vi "Mapping v10.6.3.vi"(5 "Simulate Spectra":bool, 7 "Simulate Drive":bool) -> ()   [LabVIEW 2010]
uses:
  TypeDefs/Mapping Spectra Params.ctl
  TypeDefs/Mapping Drive Params v10.6.0.ctl
  NPC3SG/TypeDefs/NPC3SG Set Positions.ctl
  NPC3SG/TypeDefs/NPC3SG Current Values.ctl
  iHR550/TypeDefs/iHR Current Values.ctl
  ITC503/TypeDefs/ITC503 Current Values.ctl
  TypeDefs/Mapping Input Parameters v10.6.2.ctl
  Symphony/TypeDefs/Symphony Area Format.ctl
  <vilib>/Utility/miscctls.llb/LVPointTypeDef.ctl
  Global Variables.vi
panel:
  in  "Input Parameters":T1={"Drive Connection Port"="", "ITC503 Current Values"={"ITC503 Heater"=0.0, "ITC503 Temperature"=0.0, "ITC503 P"=0.0, "ITC503 I"=0.0, "ITC503 D"=0.0, "ITC503 Setpoint"=0.0, "ITC503 Gradient"=0.0, "ITC503 Heater Auto"=FALSE, "ITC503 PID Auto"=FALSE}, "Wavelengths (nm)"=[], "Drive Current Values"={"Drive X Position"=0.0, "Drive Y Position"=0.0, "Drive Z Position"=0.0}, "iHR Current Values"={"iHR 550 Front Entrance"=0.0, "iHR550 Side Exit"=0.0, "iHR550 Wavelength"=897.9988, "iHR550 Exit Mirror"=2, "iHR550 Grating"="1", "Grating Index"=1}, "Spectra Settings"={"Integration Time"=1.0, "Repetitions"=1, "Mapping Spectra"=TRUE}, "CCD3500 Temperature"=0.0, "Simulate Drive"=FALSE, "Simulate Spectra"=FALSE, "JYCCDLib.IJYCCDReqd"=refnum, "CCD Area"={"XStart"=1, "YStart"=1, "XStop"=2048, "YStop"=512, "XBin"=1, "YBin"=1}, "CCD Gain"=1, "CCD ADC"=0, "Drive Calibration"=path ""} {"CCD ADC" items=["20 kHz       ", " 1 MHz       ", " 1 MHz Ultra ", "500 kHz Wrap"]; "CCD Gain" items=["High Light", "Best Dynamic Range", "High Sensitivity"]; "ITC503 Current Values"."ITC503 Gradient" format="%.2f"; "ITC503 Current Values"."ITC503 Setpoint" min=-273.0 max=300000.0 step=0.0001 format="%.1f"; "ITC503 Current Values"."ITC503 I" format="%_1f"; "ITC503 Current Values"."ITC503 P" format="%_1f"; "ITC503 Current Values"."ITC503 Temperature" min=0.0 max=1645.0 step=1e-05 format="%.2f"; "ITC503 Current Values"."ITC503 Heater" min=0.0 max=100.0 step=0.01 scale=0.0..100.0; "Drive Current Values"."Drive Z Position" min=-273.0 max=300000.0 step=0.0001 format="%.3f"; "Drive Current Values"."Drive Y Position" min=-273.0 max=300000.0 step=0.0001 format="%.3f"; "Drive Current Values"."Drive X Position" min=-273.0 max=300000.0 step=0.0001 format="%.3f"; "iHR Current Values"."iHR550 Exit Mirror" items=["EntranceMirror", "ExitMirror", "Front", "Side"]; "Spectra Settings"."Repetitions" min=1 max=100 step=1; "Spectra Settings"."Integration Time" min=0.5 max=6000.0 step=1.0 format="%.1f"}
  out "JYCCDLib.IJYCCDReqd":refnum<k7>
  out "AutoClose":bool
  out "ITC503 Temperature":dbl caption="Sample (K)" min=10.0 max=160.0 step=0.1 format="%.3f"
  out "CCD3500 Temperature":dbl caption="CCD (°C)" min=10.0 max=160.0 step=0.1 format="%.1f"
  in  "CCD Current Rep.":string="0/0"
  in  "Pause":bool
  out "Current Position":T3 {"Drive Z Position" min=-273.0 max=300000.0 step=0.0001 format="%.3f"; "Drive Y Position" min=-273.0 max=300000.0 step=0.0001 format="%.3f"; "Drive X Position" min=-273.0 max=300000.0 step=0.0001 format="%.3f"}
  out "Target Position":T7={"Drive X Set"=10.0, "Drive Y Set"=10.0, "Drive Z Set"=10.0} {"Drive X Set" min=10.0 max=160.0 step=0.1 format="%.3f"; "Drive Z Set" min=10.0 max=160.0 step=0.1 format="%.3f"; "Drive Y Set" min=10.0 max=160.0 step=0.1 format="%.3f"}
  out "Progress":u8(slide) max=10 scale=0.0..100.0
  out "Objective Running":bool caption="Obj."
  out "CCD Running":bool caption="CCD"
  in  "Save Map":bool
  in  "Spectra Params":T5={"Integration Time"=10.0, "Repetitions"=10, "Mapping Spectra"=TRUE} {"Repetitions" min=1 max=100 step=1; "Integration Time" min=0.5 max=6000.0 step=1.0 format="%.1f"}
  in  "Drive Settings":refnum<visa-resource-name>
  in  "Z Position":dbl caption="Z (µm)" min=0.0 max=100.0 step=0.1 format="%.1f"
  in  "Mapping Params":T8={"X Start Position"=0.0, "X Stop Position"=10.0, "Y Start Position"=0.0, "Y Stop Position"=10.0, "Step Size"=1.0} {"Step Size" min=0.005 max=20.0 step=0.005 format="%.3f"; "Y Stop Position" min=0.0 max=140.0 step=0.005 format="%.3f"; "Y Start Position" min=0.0 max=140.0 step=0.005 format="%.3f"; "X Stop Position" min=0.0 max=140.0 step=0.005 format="%.3f"; "X Start Position" min=0.0 max=140.0 step=0.005 format="%.3f"}
  in  "Exit":bool
  out "Measuring":bool
  in  "Start":bool
  out "Filename":string
  out "Full Data":dbl[][](array[numeric])
  out "Live Data":dbl[][](array[numeric])
  in  "ITC503 Current Values":T2 {"ITC503 Gradient" format="%.2f"; "ITC503 Setpoint" min=-273.0 max=300000.0 step=0.0001 format="%.1f"; "ITC503 I" format="%_1f"; "ITC503 P" format="%_1f"; "ITC503 Temperature" min=0.0 max=1645.0 step=1e-05 format="%.2f"; "ITC503 Heater" min=0.0 max=100.0 step=0.01 scale=0.0..100.0}
  in  "iHR Current Values":T4={"iHR 550 Front Entrance"=0.0, "iHR550 Side Exit"=0.0, "iHR550 Wavelength"=897.9988, "iHR550 Exit Mirror"=2, "iHR550 Grating"="1", "Grating Index"=1} {"iHR550 Exit Mirror" items=["EntranceMirror", "ExitMirror", "Front", "Side"]}
  in  "Wavelengths (nm)":dbl[](array[numeric])
  # "Status"
  # "Active"
  # "Target"
  # "Current"
  # "Parameters"
  # "Spectral"
  # "Spectral / Video Mapping"
  # "Mapping"
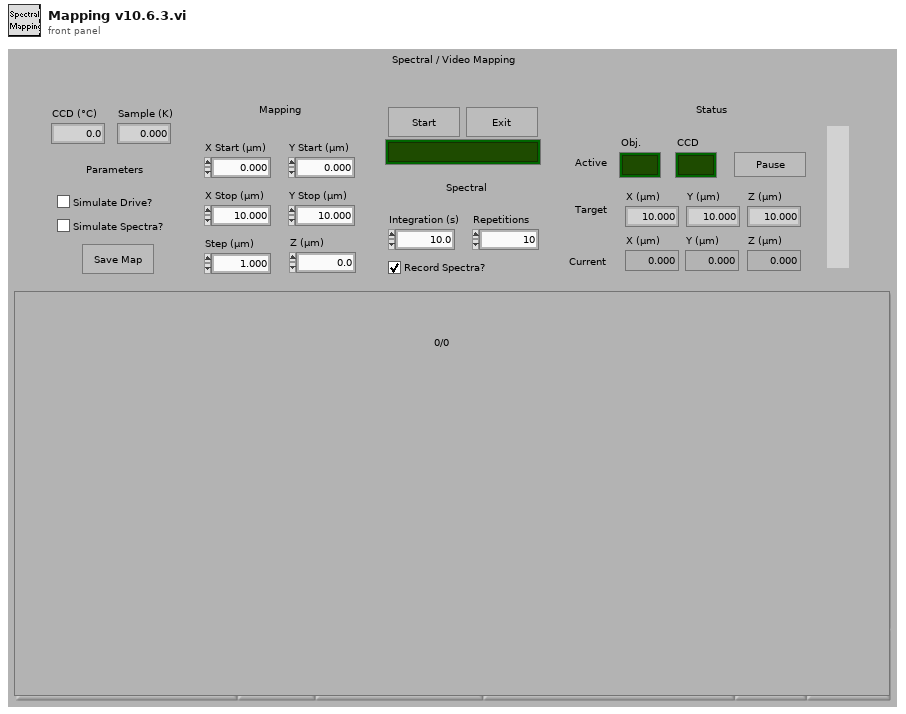
[diagram p1: front panel]
types:
  T1 = typedef "Mapping Input Parameters v10.6.2.ctl" = cluster{"Drive Connection Port":refnum<visa-resource-name>, "ITC503 Current Values":T2, "Wavelengths (nm)":dbl[], "Drive Current Values":T3, "iHR Current Values":T4, "Spectra Settings":T5, "CCD3500 Temperature":dbl, "Simulate Drive":bool, "Simulate Spectra":bool, "JYCCDLib.IJYCCDReqd":refnum<k7>, "CCD Area":T6, "CCD Gain":u16, "CCD ADC":u16, "Drive Calibration":path}
  T2 = typedef "ITC503 Current Values.ctl" = cluster{"ITC503 Heater":dbl, "ITC503 Temperature":dbl, "ITC503 P":dbl, "ITC503 I":dbl, "ITC503 D":dbl, "ITC503 Setpoint":dbl, "ITC503 Gradient":dbl, "ITC503 Heater Auto":bool, "ITC503 PID Auto":bool}
  T3 = typedef "NPC3SG Current Values.ctl" = cluster{"Drive X Position":dbl, "Drive Y Position":dbl, "Drive Z Position":dbl}
  T4 = typedef "iHR Current Values.ctl" = cluster{"iHR 550 Front Entrance":dbl, "iHR550 Side Exit":dbl, "iHR550 Wavelength":dbl, "iHR550 Exit Mirror":i32, "iHR550 Grating":string, "Grating Index":i32}
  T5 = typedef "Mapping Spectra Params.ctl" = cluster{"Integration Time":dbl, "Repetitions":u16, "Mapping Spectra":bool}
  T6 = typedef "Symphony Area Format.ctl" = cluster{"XStart":i32, "YStart":i32, "XStop":i32, "YStop":i32, "XBin":i32, "YBin":i32}
  T7 = typedef "NPC3SG Set Positions.ctl" = cluster{"Drive X Set":dbl, "Drive Y Set":dbl, "Drive Z Set":dbl}
  T8 = typedef "Mapping Drive Params v10.6.0.ctl" = cluster{"X Start Position":dbl, "X Stop Position":dbl, "Y Start Position":dbl, "Y Stop Position":dbl, "Step Size":dbl}
  T9 = typedef "LVPointTypeDef.ctl" = cluster{"Horizontal":i16, "Vertical":i16}
  T10 = cluster{"Intensities":dbl[], "Wavelengths":dbl[]}[]
  T11 = cluster{"Intensities":dbl[], "Wavelengths":dbl[]}
  T12 = enum32{"invalid app kind", "Development System", "Run Time System", "Student Edition", "Embedded LabVIEW", "Evaluation", "Custom"}
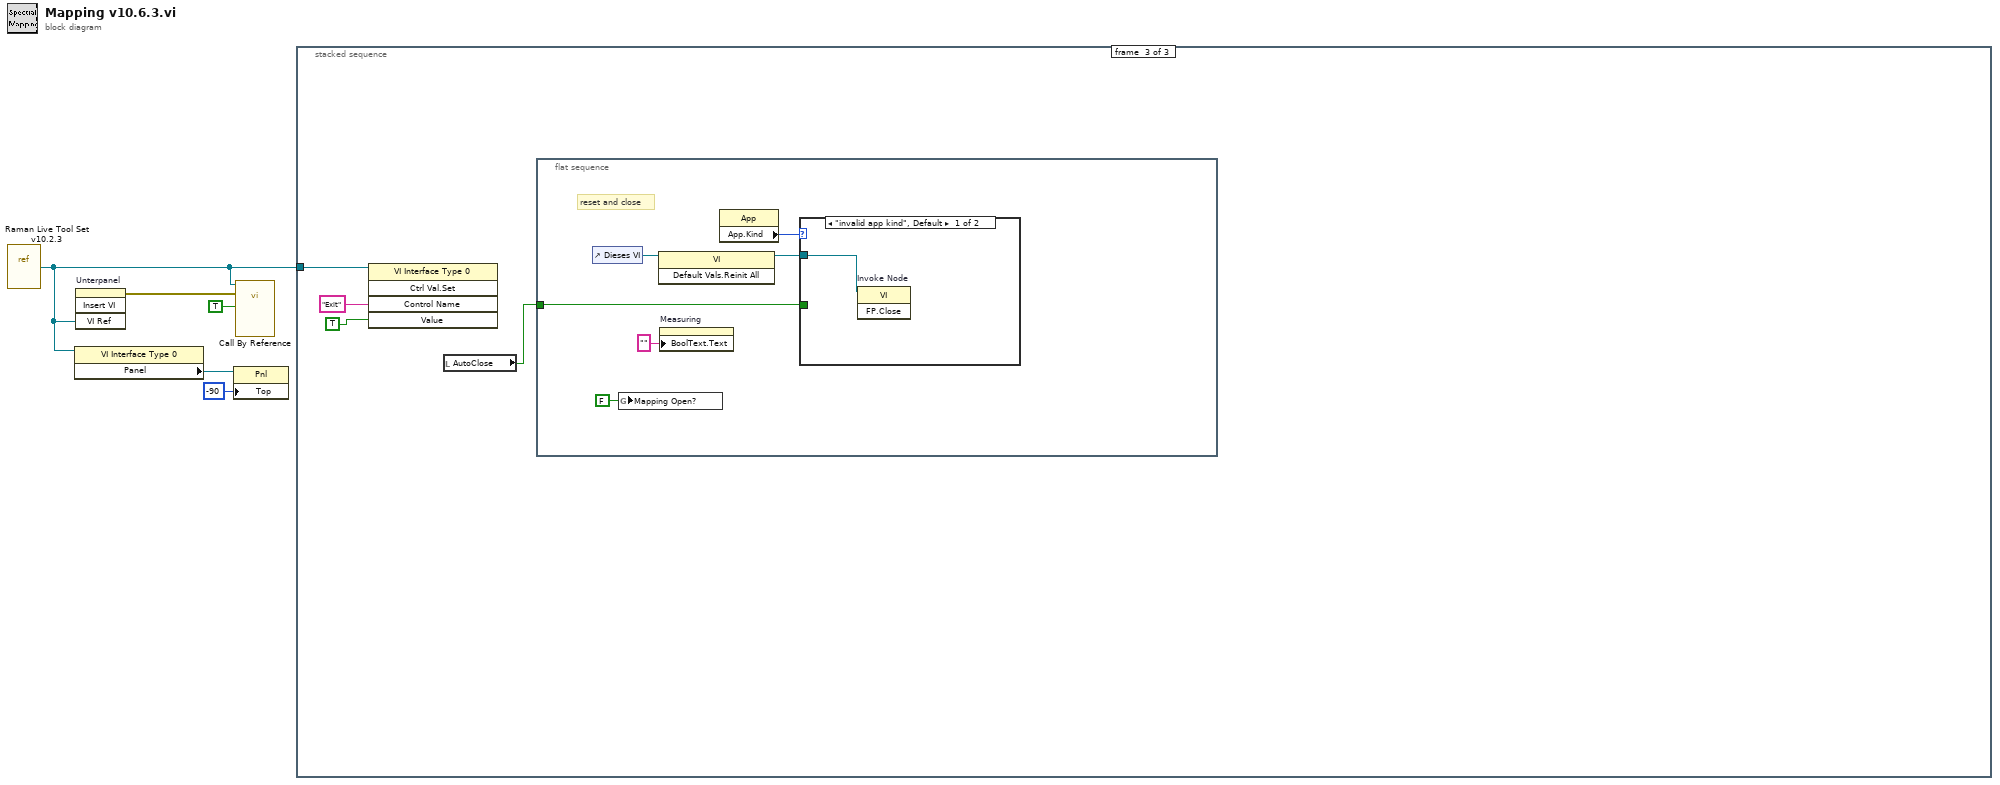
[diagram p0: block diagram]
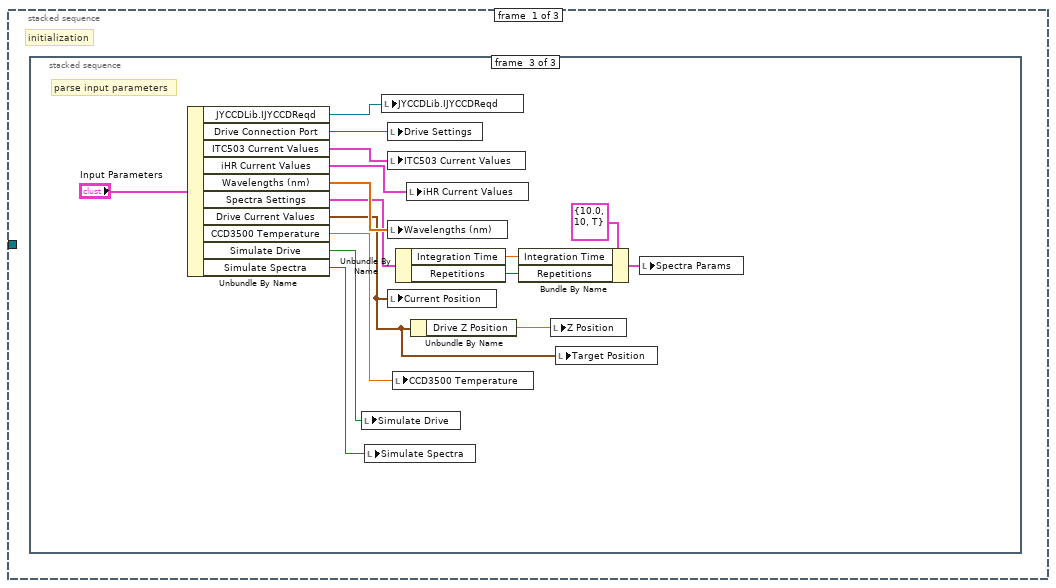
[diagram p2: hidden frame]
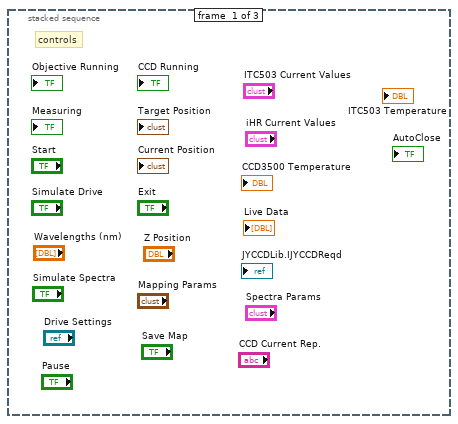
[diagram p3: hidden frame]
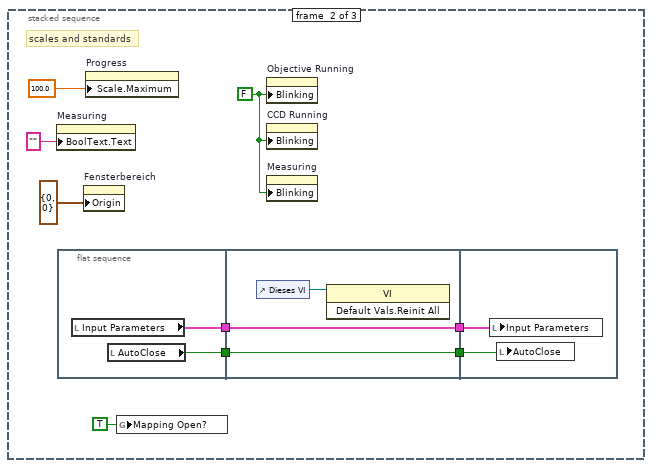
[diagram p4: hidden frame]
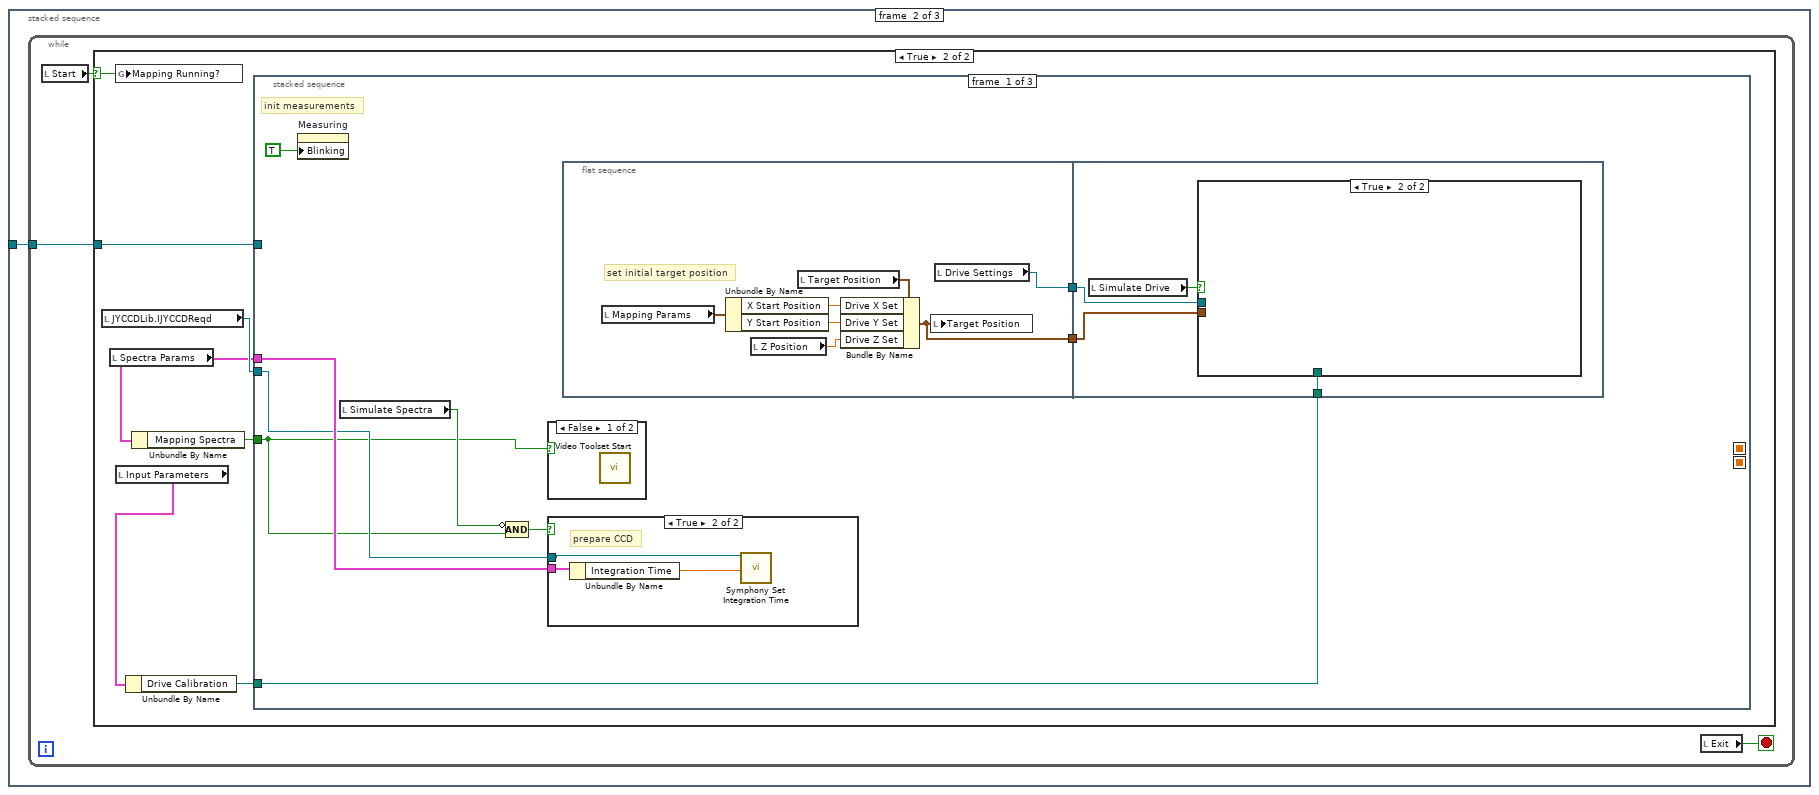
[diagram p5: hidden frame]
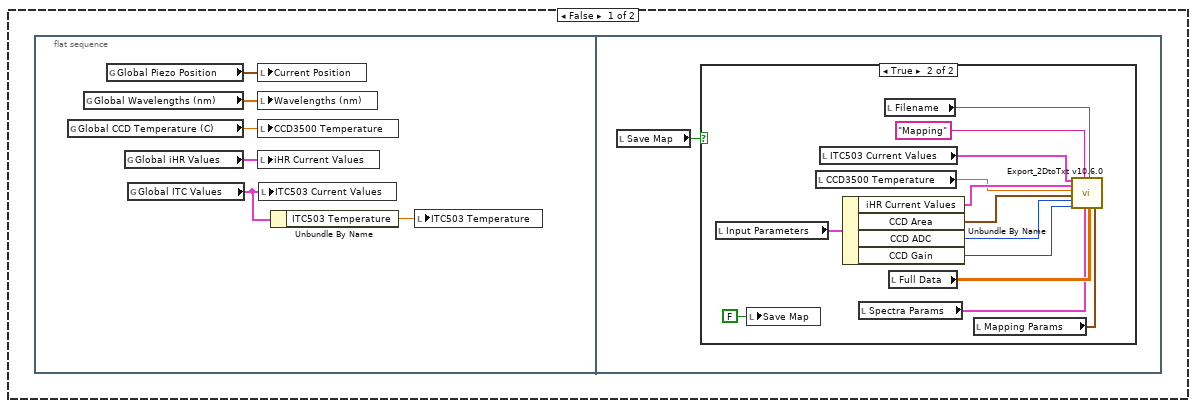
[diagram p6: hidden frame]
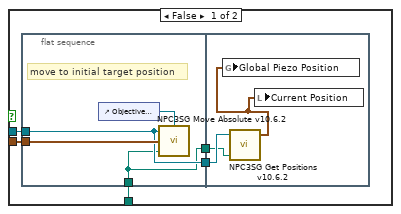
[diagram p10: hidden frame]
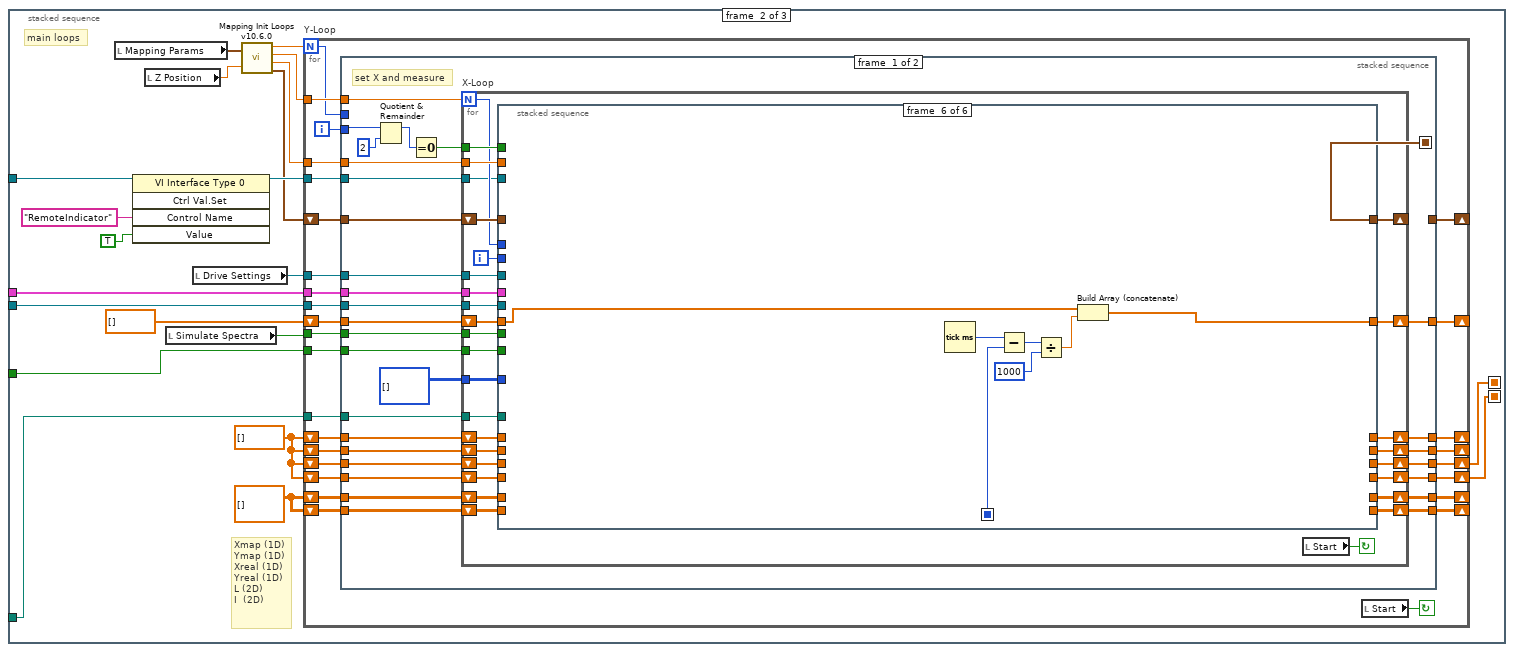
[diagram p11: hidden frame]
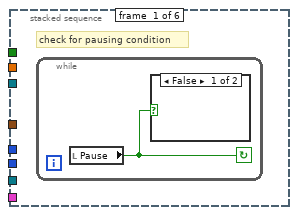
[diagram p12: hidden frame]
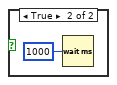
[diagram p13: hidden frame]
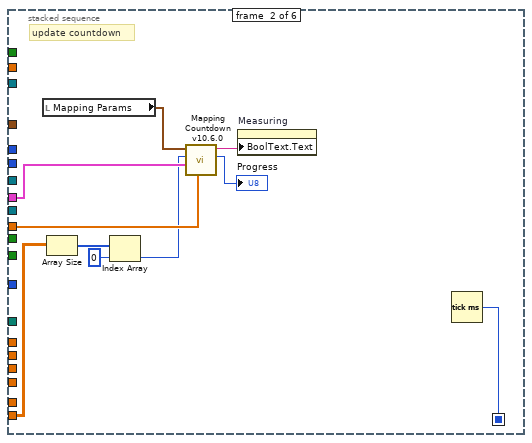
[diagram p14: hidden frame]
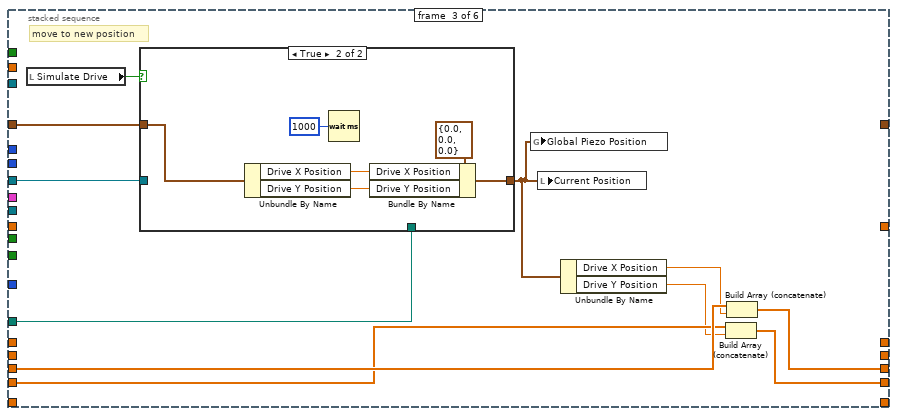
[diagram p15: hidden frame]
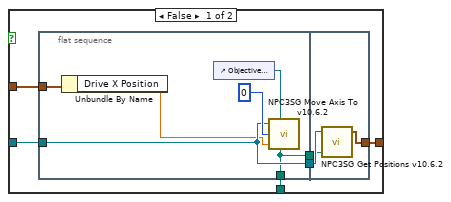
[diagram p16: hidden frame]
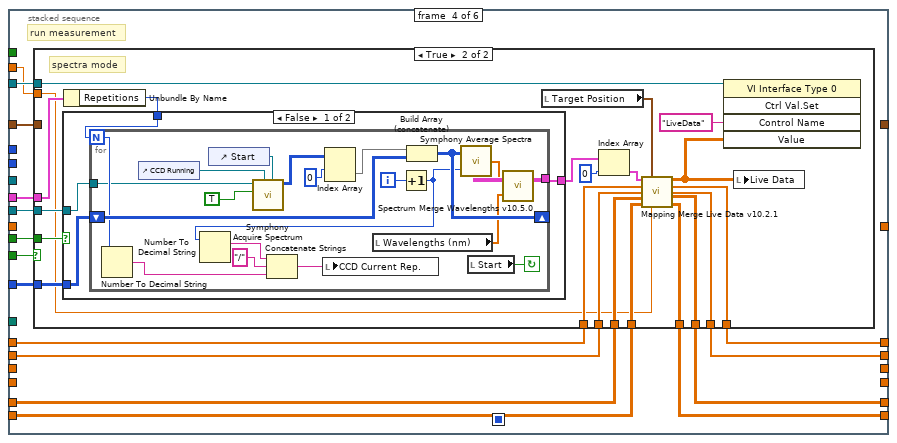
[diagram p17: hidden frame]
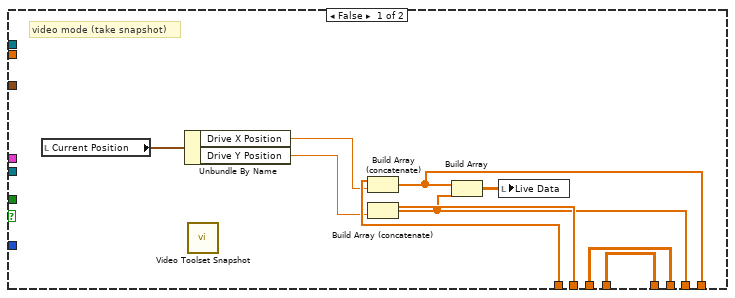
[diagram p18: hidden frame]
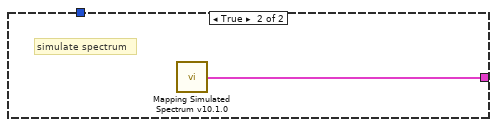
[diagram p19: hidden frame]
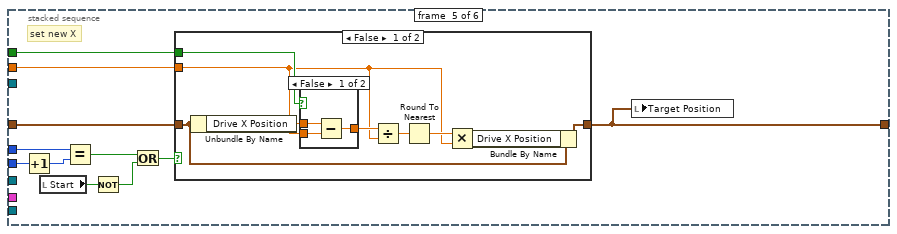
[diagram p20: hidden frame]
diagram:
  n1 = vi-ref "Raman Live Tool Set v10.2.3.vi"() -> (w3:refnum<vi>)
  n2 = property class="VI Interface Type 0"(reference=w3) -> ("Panel"=w2:refnum<vi>)  [unwired: 1 in, 2 out]
  n3 = invoke on="Unterpanel" class="Unterpanel" method="Insert VI"("VI Ref"=w3) -> (error out=w5:errorcluster)  [unwired: 3 in, 3 out]
  n4 = property class="Pnl"(reference=w2, "Top"=-90 ("Position:Oben")) -> ()  [unwired: 1 in, 2 out]
  n5 = call-by-ref "?"(reference=w3, error in=w5, "RemoteIndicator"=TRUE) -> ()  [unwired: 3 in, 2 out]
  n6 = stacked-sequence {
    tunnel: w3 -> [_ w38 w425]
    frame #0 {
      # "initialization"
      n7 = stacked-sequence {
        frame #0 {
          # "controls"
        }
        frame #1 {
          w12 = FALSE ("Blinkend")
          # "scales and standards"
          n8 = property on="Measuring" class="Bool (strict)"("BoolText.Text"="" ("Boolescher Text.Text")) -> ()  [unwired: 2 in, 2 out]
          n9 = flat-sequence {
            tunnel: [w16] -> w9
            tunnel: [w15] -> w6
            tunnel: [w18] -> w10
            tunnel: w9 -> [w18]
            tunnel: [w17] -> w7
            tunnel: w6 -> [w17]
            tunnel: w10 -> [w21]
            tunnel: w7 -> [w20]
            frame #0 {
              n10 = local read "Input Parameters"() -> (w16:T1)
              n11 = local read "AutoClose"() -> (w15:bool)
            }
            frame #1 {
              n12 = control-ref of="Dieses VI"() -> (w19:refnum<vi>)
              n13 = invoke class="VI" method="Default Vals.Reinit All"(reference=w19) -> ()  [unwired: 2 in, 3 out]
            }
            frame #2 {
              n14 = local write "Input Parameters"(w21) -> ()
              n15 = local write "AutoClose"(w20) -> ()
            }
          }
          n16 = property on="Fensterbereich" class="Pane"("Origin"=T9 {"Horizontal"=0, "Vertical"=0}) -> ()  [unwired: 2 in, 2 out]
          n17 = property on="Progress" class="Slide (strict)"("Scale.Maximum"=100.0 ("Skalierung.Bereich:Maximum")) -> ()  [unwired: 2 in, 2 out]
          n18 = global write "Global Variables.vi" "Mapping Open?"(TRUE ("Mapping Open?")) -> ()
          n19 = property on="Objective Running" class="Bool (strict)"("Blinking"=w12) -> ()  [unwired: 2 in, 2 out]
          n20 = property on="CCD Running" class="Bool (strict)"("Blinking"=w12) -> ()  [unwired: 2 in, 2 out]
          n21 = property on="Measuring" class="Bool (strict)"("Blinking"=w12) -> ()  [unwired: 2 in, 2 out]
        }
        frame #2 {
          # "parse input parameters"
          n22 = Unbundle By Name("Input Parameters") -> ("JYCCDLib.IJYCCDReqd"=w24:refnum<k7>, "Drive Connection Port"=w36:refnum<visa-resource-name>, "ITC503 Current Values"=w37:T2, "iHR Current Values"=w27:T4, "Wavelengths (nm)"=w35:dbl[], "Spectra Settings"=w33:T5, "Drive Current Values"=w22:T3, "CCD3500 Temperature"=w28:dbl, "Simulate Drive"=w26:bool, "Simulate Spectra"=w25:bool)
          n23 = local write "Simulate Drive"(w26) -> ()
          n24 = local write "Simulate Spectra"(w25) -> ()
          n25 = local write "JYCCDLib.IJYCCDReqd"(w24) -> ()
          n26 = local write "Drive Settings"(w36) -> ()
          n27 = local write "ITC503 Current Values"(w37) -> ()
          n28 = local write "Wavelengths (nm)"(w35) -> ()
          n29 = local write "Current Position"(w22) -> ()
          n30 = local write "CCD3500 Temperature"(w28) -> ()
          n31 = Unbundle By Name(w33) -> ("Integration Time"=w31:dbl, "Repetitions"=w30:u16)
          n32 = local write "iHR Current Values"(w27) -> ()
          n33 = Unbundle By Name(w22) -> ("Drive Z Position"=w34:dbl)
          n34 = Bundle By Name(cluster=T5 {"Integration Time"=10.0, "Repetitions"=10, "Mapping Spectra"=TRUE} ("Mapping Spectra Settings"), "Integration Time"=w31, "Repetitions"=w30) -> (w29:T5)
          n35 = local write "Z Position"(w34) -> ()
          n36 = local write "Target Position"(w22) -> ()
          n37 = local write "Spectra Params"(w29) -> ()
        }
      }
    }
    frame #1 {
      n38 = while {
        tunnel: w38 -> [w41]
        stop <- w40 stop-if-true
        n39 = local read "Start"() -> (w39:bool)
        n40 = case shown="True" w39 {
          selector: w39 -> [_ w65]
          tunnel: w41 -> [_ w68]
          frame False {
            n41 = flat-sequence {
              frame #0 {
                n42 = global read "Global Variables.vi" "Global CCD Temperature (C)"() -> (w47:dbl)
                n43 = global read "Global Variables.vi" "Global Wavelengths (nm)"() -> (w45:dbl[])
                n44 = global read "Global Variables.vi" "Global Piezo Position"() -> (w46:T3)
                n45 = global read "Global Variables.vi" "Global iHR Values"() -> (w44:T4)
                n46 = global read "Global Variables.vi" "Global ITC Values"() -> (w43:T2)
                n47 = local write "Current Position"(w46) -> ()
                n48 = local write "Wavelengths (nm)"(w45) -> ()
                n49 = local write "CCD3500 Temperature"(w47) -> ()
                n50 = local write "iHR Current Values"(w44) -> ()
                n51 = local write "ITC503 Current Values"(w43) -> ()
                n52 = Unbundle By Name(w43) -> ("ITC503 Temperature"=w42:dbl)
                n53 = local write "ITC503 Temperature"(w42) -> ()
              }
              frame #1 {
                n54 = local read "Save Map"() -> (w48:bool)
                n55 = case shown="True" w48 {
                  frame False {
                  }
                  frame True {
                    n56 = local read "Input Parameters"() -> (w57:T1)
                    n57 = local write "Save Map"(FALSE ("Save Map")) -> ()
                    n58 = local read "CCD3500 Temperature"() -> (w51:dbl)
                    n59 = local read "ITC503 Current Values"() -> (w54:T2)
                    n60 = Unbundle By Name(w57) -> ("iHR Current Values"=w52:T4, "CCD Area"=w53:T6, "CCD ADC"=w56:u16, "CCD Gain"=w55:u16)
                    n61 = local read "Spectra Params"() -> (w50:T5)
                    n62 = local read "Filename"() -> (w60:string)
                    n63 = local read "Full Data"() -> (w58:dbl[][])
                    n64 = local read "Mapping Params"() -> (w49:T8)
                    n65 = call "Export_2DtoTxt v10.6.0.vi"("ITC503 Current Values"=w54, "iHR Current Values"=w52, "CCD Temperature"=w51, "CCD Area"=w53, "CCD ADC"=w56, "CCD Gain"=w55, "Export Type"="Mapping", "Spectra Settings"=w50, "Filename"=w60, "Data (2D)"=w58, "Mapping Parameters"=w49) -> ()  [unwired: 8 in, 1 out]
                  }
                }
              }
            }
          }
          frame True {
            n66 = local read "JYCCDLib.IJYCCDReqd"() -> (w67:refnum<k7>)
            n67 = local read "Spectra Params"() -> (w66:T5)
            n68 = global write "Global Variables.vi" "Mapping Running?"(w65) -> ()
            n69 = local read "Input Parameters"() -> (w63:T1)
            n70 = Unbundle By Name(w63) -> ("Drive Calibration"=w62:path)
            n71 = Unbundle By Name(w66) -> ("Mapping Spectra"=w64:bool)
            n72 = stacked-sequence {
              seq-local: [_ w105 _] -> [_ _ w400]
              seq-local: [_ w106 _] -> [_ _ w399]
              tunnel: w68 -> [_ w116 _]
              tunnel: w64 -> [w70 w115 w401]
              tunnel: w66 -> [w72 w113 _]
              tunnel: w67 -> [w71 w112 _]
              tunnel: w62 -> [w69 w104 _]
              frame #0 {
                # "init measurements"
                n73 = property on="Measuring" class="Bool (strict)"("Blinking"=TRUE ("Blinkend")) -> ()  [unwired: 2 in, 2 out]
                n74 = local read "Simulate Spectra"() -> (w74:bool)
                n75 = Compound Arithmetic op=AND(invert w74, w70) -> (w73:bool)
                n76 = case shown="False" w70 {
                  frame False {
                    n77 = call "Video Toolset Start.vi"() -> ()  [unwired: 3 in]
                  }
                  frame True {
                  }
                }
                n78 = case shown="True" w73 {
                  tunnel: w71 -> [_ w80]
                  tunnel: w72 -> [_ w79]
                  frame False {
                  }
                  frame True {
                    # "prepare CCD"
                    n79 = Unbundle By Name(w79) -> ("Integration Time"=w78:dbl)
                    n80 = call "Symphony Set Integration Time.vi"("JYCCDLib.IJYCCDReqd"=w80, "Integration (s)"=w78) -> ()  [unwired: 13 in, 1 out]
                  }
                }
                n81 = flat-sequence {
                  tunnel: [w82] -> w76
                  tunnel: [w81] -> w75
                  tunnel: w76 -> [w89]
                  tunnel: w75 -> [w90]
                  tunnel: w69 -> [w88]
                  frame #0 {
                    # "set initial target position"
                    n82 = local read "Mapping Params"() -> (w87:T8)
                    n83 = Unbundle By Name(w87) -> ("X Start Position"=w85:dbl, "Y Start Position"=w84:dbl)
                    n84 = local read "Z Position"() -> (w83:dbl)
                    n85 = local read "Target Position"() -> (w86:T7)
                    n86 = Bundle By Name(cluster=w86, "Drive X Set"=w85, "Drive Y Set"=w84, "Drive Z Set"=w83) -> (w82:T7)
                    n87 = local write "Target Position"(w82) -> ()
                    n88 = local read "Drive Settings"() -> (w81:refnum<visa-resource-name>)
                  }
                  frame #1 {
                    n89 = local read "Simulate Drive"() -> (w91:bool)
                    n90 = case shown="True" w91 {
                      tunnel: w90 -> [w96 _]
                      tunnel: w89 -> [w94 _]
                      tunnel: w88 -> [w93 _]
                      frame False {
                        n91 = flat-sequence {
                          tunnel: w96 -> [w98]
                          tunnel: [w98] -> w95
                          tunnel: w94 -> [w99]
                          tunnel: w93 -> [w97]
                          tunnel: [w97] -> w92
                          tunnel: w95 -> [w102]
                          tunnel: w92 -> [w101]
                          frame #0 {
                            # "move to initial target position"
                            n92 = control-ref of="Objective Running"() -> (w100:refnum<vi>)
                            n93 = call "NPC3SG Move Absolute v10.6.2.vi"("Running"=w100, "Calibration File"=w97, "Drive New Abs. Positions"=w99, "Drive Visa Name"=w98) -> ()  [unwired: 1 in]
                          }
                          frame #1 {
                            n94 = call "NPC3SG Get Positions v10.6.2.vi"("Drive Visa Name"=w102, "Calibration File"=w101) -> ("Drive Current Values"=w103:T3)  [unwired: 5 in]
                            n95 = global write "Global Variables.vi" "Global Piezo Position"(w103) -> ()
                            n96 = local write "Current Position"(w103) -> ()
                          }
                        }
                      }
                      frame True {
                      }
                    }
                  }
                }
              }
              frame #1 {
                w124 = dbl[][] []
                w107 = dbl[] []
                # "main loops"
                # "Xmap (1D)\nYmap (1D)\nXreal (1D)\nYreal (1D)\nL (2D)\nI  (2D)"
                n97 = local read "Mapping Params"() -> (w110:T8)
                n98 = invoke class="VI Interface Type 0" method="Ctrl Val.Set"(reference=w116, "Control Name"="RemoteIndicator" ("Elementname"), "Value"=TRUE) -> (reference out=w118:refnum<vi>)  [unwired: 2 in, 4 out]
                n99 = local read "Z Position"() -> (w109:dbl)
                n100 = local read "Simulate Spectra"() -> (w108:bool)
                n101 = local read "Drive Settings"() -> (w111:refnum<visa-resource-name>)
                n102 = call "Mapping Init Loops v10.6.0.vi"("Z Position"=w109, "Mapping Params"=w110) -> ("Start Positions"=w117:T3, "Step Size"=w119:dbl, "X Steps"=w120:dbl, "Y Steps"=w121:dbl)
                n103 = for "Y-Loop" {
                  N: w121 -> [w138]
                  tunnel: w120 -> [w151]
                  tunnel: w119 -> [w150]
                  shift-right: [w136] -> _
                  shift-left: w117 -> [w137]
                  shift-right: [w142] -> _
                  shift-left: w124 -> [w146]
                  shift-right: [w143] -> _
                  shift-left: w124 -> [w147]
                  shift-right: [w145] -> _
                  shift-left: w107 -> [w149]
                  shift-right: [w144] -> _
                  shift-left: w107 -> [w148]
                  tunnel: w118 -> [w140]
                  tunnel: w108 -> [w139]
                  tunnel: w111 -> [w135]
                  tunnel: w115 -> [w134]
                  tunnel: w113 -> [w133]
                  shift-right: [w131] -> _
                  shift-left: dbl[] [] -> [w132]
                  tunnel: w112 -> [w130]
                  shift-right: [w127] -> w106
                  shift-left: w107 -> [w128]
                  shift-right: [w126] -> w105
                  shift-left: w107 -> [w129]
                  tunnel: w104 -> [w125]
                  i -> [w141]
                  stop <- w152 continue-if-true
                  n104 = stacked-sequence {
                    seq-local: [w167 _] -> [_ w370]
                    tunnel: w151 -> [w182 _]
                    tunnel: w150 -> [w181 w371]
                    tunnel: w149 -> [w180 _]
                    tunnel: w148 -> [w179 _]
                    tunnel: w147 -> [w178 _]
                    tunnel: w146 -> [w154 _]
                    tunnel: [w177 _] -> w145
                    tunnel: [w176 _] -> w144
                    tunnel: [w175 _] -> w143
                    tunnel: [w174 _] -> w142
                    tunnel: w141 -> [w171 w374]
                    tunnel: w140 -> [w169 _]
                    tunnel: w139 -> [w168 _]
                    tunnel: w138 -> [_ w372]
                    tunnel: w137 -> [w166 _]
                    tunnel: [_ w368] -> w136
                    tunnel: w135 -> [w165 w369]
                    tunnel: w134 -> [w164 _]
                    tunnel: w133 -> [w163 _]
                    tunnel: w132 -> [w162 _]
                    tunnel: [w161 _] -> w131
                    tunnel: w130 -> [w160 _]
                    tunnel: w129 -> [w158 _]
                    tunnel: w128 -> [w157 _]
                    tunnel: [w156 _] -> w127
                    tunnel: [w155 _] -> w126
                    tunnel: w125 -> [w153 w362]
                    frame #0 {
                      # "set X and measure"
                      n105 = Quotient & Remainder(x=w171, y=2) -> (x-y*floor(x/y)=w172:i32)  [unwired: 1 out]
                      n106 = Equal To 0?(x=w172) -> (x = 0?=w170:bool)
                      n107 = for "X-Loop" {
                        N: w182 -> [w197]
                        tunnel: w181 -> [w209]
                        shift-right: [w208] -> w167
                        shift-left: w166 -> [w210]
                        shift-right: [w203] -> w177
                        shift-left: w180 -> [w207]
                        shift-right: [w202] -> w176
                        shift-left: w179 -> [w206]
                        shift-right: [w200] -> w175
                        shift-left: w178 -> [w205]
                        shift-right: [w201] -> w174
                        shift-left: w154 -> [w204]
                        tunnel: w170 -> [w199]
                        tunnel: w169 -> [w196]
                        tunnel: w168 -> [w195]
                        tunnel: w165 -> [w194]
                        tunnel: w164 -> [w193]
                        tunnel: w163 -> [w192]
                        shift-right: [w191] -> w161
                        shift-left: w162 -> [w190]
                        tunnel: w160 -> [w189]
                        tunnel: u16[][] [] -> [w188]
                        shift-right: [w184] -> w155
                        shift-left: w158 -> [w187]
                        shift-right: [w185] -> w156
                        shift-left: w157 -> [w186]
                        tunnel: w153 -> [w183]
                        i -> [w198]
                        stop <- w211 continue-if-true
                        n108 = stacked-sequence {
                          seq-local: [_ w218 _ _ _ _] -> [_ _ _ _ _ w358]
                          tunnel: w210 -> [_ _ w234 w271 w335 _]
                          tunnel: w209 -> [_ _ _ w256 w333 _]
                          tunnel: [_ _ _ _ w332 _] -> w208
                          tunnel: w207 -> [_ _ _ w270 _ _]
                          tunnel: w206 -> [_ _ _ w269 _ _]
                          tunnel: w205 -> [_ _ _ w267 _ _]
                          tunnel: w204 -> [_ w217 _ w268 _ _]
                          tunnel: [_ _ _ w266 _ _] -> w203
                          tunnel: [_ _ _ w265 _ _] -> w202
                          tunnel: [_ _ _ w264 _ _] -> w201
                          tunnel: [_ _ _ w263 _ _] -> w200
                          tunnel: w199 -> [_ _ _ _ w334 _]
                          tunnel: w198 -> [_ _ _ _ w338 _]
                          tunnel: w197 -> [_ _ _ _ w336 _]
                          tunnel: w196 -> [_ _ _ w262 _ _]
                          tunnel: w195 -> [_ _ _ w261 _ _]
                          tunnel: w194 -> [_ _ w232 _ _ _]
                          tunnel: w193 -> [_ _ _ w260 _ _]
                          tunnel: w192 -> [_ w220 _ w258 _ _]
                          tunnel: [_ _ _ _ _ w355] -> w191
                          tunnel: w190 -> [_ w219 _ _ _ w357]
                          tunnel: w189 -> [_ _ _ w259 _ _]
                          tunnel: w188 -> [_ _ _ w257 _ _]
                          tunnel: w187 -> [_ _ w231 _ _ _]
                          tunnel: w186 -> [_ _ w230 _ _ _]
                          tunnel: [_ _ w227 _ _ _] -> w185
                          tunnel: [_ _ w226 _ _ _] -> w184
                          tunnel: w183 -> [_ _ w224 _ _ _]
                          frame #0 {
                            # "check for pausing condition"
                            n109 = while {
                              stop <- w212 continue-if-true
                              n110 = local read "Pause"() -> (w212:bool)
                              n111 = case shown="False" w212 {
                                frame False {
                                }
                                frame True {
                                n112 = Wait (ms)(milliseconds to wait=u32 1000) -> ()  [unwired: 1 out]
                                }
                              }
                            }
                          }
                          frame #1 {
                            # "update countdown"
                            n113 = local read "Mapping Params"() -> (w223:T8)
                            n114 = Array Size(array=w217) -> (size(s)=w216:i32[])
                            n115 = Index Array(array=w216, index=0) -> (element=w214:i32)
                            n116 = call "Mapping Countdown v10.6.0.vi"("Execution Times (s)"=w219, "Mapping Spectra Settings"=w220, "Ready Steps"=w214, "Mapping Drive Parameters"=w223) -> ("Progress"=→"Progress":i16, "Time String"=w221:string)  [unwired: 6 in]
                            n117 = property on="Measuring" class="Bool (strict)"("BoolText.Text"=w221) -> ()  [unwired: 2 in, 2 out]
                            n118 = Tick Count (ms)() -> (millisecond timer value=w218:u32)
                          }
                          frame #2 {
                            # "move to new position"
                            n119 = local read "Simulate Drive"() -> (w233:bool)
                            n120 = case shown="True" w233 {
                              tunnel: w234 -> [w240 w254]
                              tunnel: w232 -> [w239 _]
                              tunnel: [w237 w250] -> w225
                              tunnel: w224 -> [w236 _]
                              frame False {
                                n121 = flat-sequence {
                                tunnel: w240 -> [w243]
                                tunnel: w239 -> [w244]
                                tunnel: [w244] -> w238
                                tunnel: w236 -> [w241]
                                tunnel: [w241] -> w235
                                tunnel: w238 -> [w249]
                                tunnel: [w248] -> w237
                                tunnel: w235 -> [w247]
                                frame #0 {
                                n122 = Unbundle By Name(w243) -> ("Drive X Position"=w242:dbl)
                                n123 = control-ref of="Objective Running"() -> (w245:refnum<vi>)
                                n124 = call "NPC3SG Move Axis To v10.6.2.vi"("Drive Visa Name"=w244, "Running"=w245, "Axis"=0, "Drive Set"=w242, "Calibration File"=w241) -> ()  [unwired: 2 in, 1 out]
                                }
                                frame #1 {
                                n125 = call "NPC3SG Get Positions v10.6.2.vi"("Drive Visa Name"=w249, "Calibration File"=w247) -> ("Drive Current Values"=w248:T3)  [unwired: 5 in]
                                }
                                }
                              }
                              frame True {
                                n126 = Unbundle By Name(w254) -> ("Drive X Position"=w255:dbl, "Drive Y Position"=w252:dbl)
                                n127 = Wait (ms)(milliseconds to wait=u32 1000 ("Zu wartende ms")) -> ()  [unwired: 1 out]
                                n128 = Bundle By Name(cluster=T3 {"Drive X Position"=0.0, "Drive Y Position"=0.0, "Drive Z Position"=0.0} ("Drive Current Values"), "Drive X Position"=w255, "Drive Y Position"=w252) -> (w250:T3)
                              }
                            }
                            n129 = global write "Global Variables.vi" "Global Piezo Position"(w225) -> ()
                            n130 = local write "Current Position"(w225) -> ()
                            n131 = Unbundle By Name(w225) -> ("Drive X Position"=w229:dbl, "Drive Y Position"=w228:dbl)
                            n132 = Build Array (concatenate)(w230, w228) -> (w227:dbl[])
                            n133 = Build Array (concatenate)(w231, w229) -> (w226:dbl[])
                          }
                          frame #3 {
                            # "run measurement"
                            n134 = case shown="True" w260 {
                              tunnel: w271 -> [_ _]
                              tunnel: w270 -> [w278 w299]
                              tunnel: w269 -> [w277 w298]
                              tunnel: w268 -> [w280 w296]
                              tunnel: w267 -> [w281 w297]
                              tunnel: [w275 w293] -> w266
                              tunnel: [w276 w292] -> w265
                              tunnel: [w280 w295] -> w264
                              tunnel: [w281 w294] -> w263
                              tunnel: w262 -> [_ w301]
                              tunnel: w261 -> [_ w300]
                              tunnel: w259 -> [_ w289]
                              tunnel: w258 -> [_ w288]
                              tunnel: w257 -> [_ w286]
                              tunnel: w256 -> [_ w282]
                              frame False {
                                # "video mode (take snapshot)"
                                n135 = local read "Current Position"() -> (w279:T3)
                                n136 = Unbundle By Name(w279) -> ("Drive X Position"=w274:dbl, "Drive Y Position"=w273:dbl)
                                n137 = call "Video Toolset Snapshot.vi"() -> ()  [unwired: 12 in]
                                n138 = Build Array (concatenate)(w278, w274) -> (w275:dbl[])
                                n139 = Build Array (concatenate)(w277, w273) -> (w276:dbl[])
                                n140 = Build Array(w275, w276) -> (w272:dbl[][])
                                n141 = local write "Live Data"(w272) -> ()
                              }
                              frame True {
                                # "spectra mode"
                                n142 = Unbundle By Name(w288) -> ("Repetitions"=w287:u16)
                                n143 = case shown="False" w300 {
                                tunnel: [w305 w327] -> w285
                                tunnel: w289 -> [w306 _]
                                tunnel: w287 -> [w304 _]
                                tunnel: w286 -> [w303 _]
                                frame False {
                                n144 = for {
                                N: w304 -> [w313]
                                shift-right: [w324] -> _
                                shift-left: w303 -> [w325]
                                tunnel: [w322] -> w305
                                tunnel: w306 -> [w311]
                                i -> [w326]
                                stop <- w320 continue-if-true
                                n145 = Number To Decimal String(number=w313) -> (decimal integer string=w316:string)  [unwired: 1 in]
                                n146 = control-ref of="CCD Running"() -> (w319:refnum<vi>)
                                n147 = control-ref of="Start"() -> (w318:refnum<vi>)
                                n148 = call "Symphony Acquire Spectrum.vi"("Acquire"=w318, "Running"=w319, "ShutterOpen"=TRUE, "JYCCDLib.IJYCCDReqd"=w311) -> ("Raw Data"=w308:i32[][])  [unwired: 6 in, 1 out]
                                n149 = Index Array(array=w308, index (row)=0) -> (element=w307:i32[])  [unwired: 1 in]
                                n150 = local read "Wavelengths (nm)"() -> (w321:dbl[])
                                n151 = Increment(x=w326) -> (x+1=w312:i32)
                                n152 = Number To Decimal String(number=w312) -> (decimal integer string=w315:string)  [unwired: 1 in]
                                n153 = Concatenate Strings(w315, "/" ("string"), w316) -> (w314:string)
                                n154 = local write "CCD Current Rep."(w314) -> ()
                                n155 = Build Array (concatenate)(w307, w325) -> (w324:i32[][])
                                n156 = call "Symphony Average Spectra.vi"("Repetitions"=w312, "Raw Spectra"=w324) -> ("Raw Spectrum"=w323:dbl[])
                                n157 = local read "Start"() -> (w320:bool)
                                n158 = call "Spectrum Merge Wavelengths v10.5.0.vi"("Wavelengths (nm)"=w321, "Raw Spectrum"=w323) -> ("Spectrum-Cluster"=w322:T10)  [unwired: 1 out]
                                }
                                }
                                frame True {
                                # "simulate spectrum"
                                n159 = call "Mapping Simulated Spectrum v10.1.0.vi"() -> ("Simulated Spectrum"=w327:cluster{i32[], dbl[]}[])
                                }
                                }
                                n160 = local read "Target Position"() -> (w291:T7)
                                n161 = Index Array(array=w285, index=0 ("Index")) -> (element=w284:T11)
                                n162 = call "Mapping Merge Live Data v10.2.1.vi"("New Spectrum"=w284, "Target Position"=w291, "X in (1D)"=w299, "Y in (1D)"=w298, "L in (2D)"=w297, "I in (2D)"=w296, "Step Size"=w282) -> ("Live Data"=w290:dbl[][], "X out (1D)"=w293:dbl[], "Y out (1D)"=w292:dbl[], "L out (2D)"=w294:dbl[][], "I out (2D)"=w295:dbl[][])  [unwired: 4 in]
                                n163 = invoke class="VI Interface Type 0" method="Ctrl Val.Set"(reference=w301, "Control Name"="LiveData" ("Elementname"), "Value"=w290) -> ()  [unwired: 2 in, 5 out]
                                n164 = local write "Live Data"(w290) -> ()
                              }
                            }
                          }
                          frame #4 {
                            # "set new X"
                            n165 = Increment(x=w338) -> (x+1=w337:i32)
                            n166 = local read "Start"() -> (w331:bool)
                            n167 = Equal?(x=w336, y=w337) -> (x = y?=w328:bool)
                            n168 = Not(x=w331) -> (.not. x?=w330:bool)
                            n169 = Or(x=w328, y=w330) -> (x .or. y?=w329:bool)
                            n170 = case shown="False" w329 {
                              tunnel: w335 -> [w346 w354]
                              tunnel: [w345 w354] -> w332
                              tunnel: w334 -> [w344 _]
                              tunnel: w333 -> [w339 _]
                              frame False {
                                n171 = Unbundle By Name(w346) -> ("Drive X Position"=w347:dbl)
                                n172 = case shown="False" w344 {
                                tunnel: w347 -> [w350 w352]
                                tunnel: [w349 w353] -> w340
                                tunnel: w339 -> [w348 w351]
                                frame False {
                                n173 = Subtract(x=w350, y=w348) -> (x-y=w349:dbl)
                                }
                                frame True {
                                n174 = Add(x=w352, y=w351) -> (x+y=w353:dbl)
                                }
                                }
                                n175 = Divide(x=w340, y=w339) -> (x/y=w343:dbl)
                                n176 = Round To Nearest(number=w343) -> (nearest integer value=w342:dbl)
                                n177 = Multiply(x=w342, y=w339) -> (x*y=w341:dbl)
                                n178 = Bundle By Name(cluster=w346, "Drive X Position"=w341) -> (w345:T3)
                              }
                              frame True {
                              }
                            }
                            n179 = local write "Target Position"(w332) -> ()
                          }
                          frame #5 {
                            n180 = Tick Count (ms)() -> (millisecond timer value=w359:u32)
                            n181 = Subtract(x=w359, y=w358) -> (x-y=w361:u32)
                            n182 = Divide(x=w361, y=u32 1000) -> (x/y=w356:dbl)
                            n183 = Build Array (concatenate)(w357, w356) -> (w355:dbl[])
                          }
                        }
                        n184 = local read "Start"() -> (w211:bool)
                      }
                    }
                    frame #1 {
                      # "set new Y\nand move to new position"
                      n185 = Increment(x=w374) -> (x+1=w373:i32)
                      n186 = local read "Start"() -> (w364:bool)
                      n187 = Equal?(x=w372, y=w373) -> (x = y?=w366:bool)
                      n188 = local read "Simulate Drive"() -> (w367:bool)
                      n189 = Not(x=w364) -> (.not. x?=w365:bool)
                      n190 = Or(x=w366, y=w365) -> (x .or. y?=w363:bool)
                      n191 = case shown="False" w363 {
                        tunnel: w370 -> [w397 w398]
                        tunnel: [w396 w398] -> w368
                        tunnel: w371 -> [w391 _]
                        frame False {
                          n192 = Unbundle By Name(w397) -> ("Drive Y Position"=w395:dbl)
                          n193 = Add(x=w391, y=w395) -> (x+y=w392:dbl)
                          n194 = Divide(x=w392, y=w391) -> (x/y=w393:dbl)
                          n195 = Round To Nearest(number=w393) -> (nearest integer value=w394:dbl)
                          n196 = Multiply(x=w394, y=w391) -> (x*y=w390:dbl)
                          n197 = Bundle By Name(cluster=w397, "Drive Y Position"=w390) -> (w396:T3)
                        }
                        frame True {
                        }
                      }
                      n198 = case shown="True" w367 {
                        tunnel: w369 -> [w379 _]
                        tunnel: w368 -> [w378 _]
                        tunnel: w362 -> [w376 _]
                        frame False {
                          n199 = flat-sequence {
                            tunnel: w379 -> [w385]
                            tunnel: w378 -> [w384]
                            tunnel: [w385] -> w380
                            tunnel: w376 -> [w381]
                            tunnel: [w381] -> w375
                            tunnel: [w389] -> w377
                            tunnel: w380 -> [w388]
                            tunnel: w375 -> [w387]
                            frame #0 {
                              n200 = Unbundle By Name(w384) -> ("Drive Y Position"=w383:dbl)
                              n201 = control-ref of="Objective Running"() -> (w386:refnum<vi>)
                              n202 = call "NPC3SG Move Axis To v10.6.2.vi"("Drive Visa Name"=w385, "Running"=w386, "Axis"=1, "Drive Set"=w383, "Calibration File"=w381) -> ()  [unwired: 2 in, 1 out]
                            }
                            frame #1 {
                              n203 = call "NPC3SG Get Positions v10.6.2.vi"("Drive Visa Name"=w388, "Calibration File"=w387) -> ("Drive Current Values"=w389:T3)  [unwired: 5 in]
                            }
                          }
                          n204 = global write "Global Variables.vi" "Global Piezo Position"(w377) -> ()
                          n205 = local write "Current Position"(w377) -> ()
                        }
                        frame True {
                        }
                      }
                      n206 = local write "Target Position"(w368) -> ()
                    }
                  }
                  n207 = local read "Start"() -> (w152:bool)
                }
              }
              frame #2 {
                # "conclude measurement"
                n208 = flat-sequence {
                  tunnel: w400 -> [w413]
                  tunnel: w399 -> [w412]
                  tunnel: w401 -> [w418]
                  frame #0 {
                    # "save data"
                    n209 = local read "Input Parameters"() -> (w406:T1)
                    n210 = global read "Global Variables.vi" "Global iHR Values"() -> (w409:T4)
                    n211 = global read "Global Variables.vi" "Global ITC Values"() -> (w410:T2)
                    n212 = local read "Spectra Params"() -> (w407:T5)
                    n213 = global read "Global Variables.vi" "Global CCD Temperature (C)"() -> (w408:dbl)
                    n214 = Unbundle By Name(w406) -> ("CCD Area"=w405:T6, "CCD Gain"=w403:u16, "CCD ADC"=w404:u16)
                    n215 = local read "Mapping Params"() -> (w402:T8)
                    n216 = call "Export_mappingFileName v10.5.1.vi"("ITC503 Current Values"=w410, "iHR Current Values"=w409, "Spectra Settings"=w407, "Mapping Parameters"=w402) -> ("Filename"=w416:string)  [unwired: 1 in]
                    "Filename" <- w416
                    n217 = local read "Live Data"() -> (w415:dbl[][])
                    n218 = Unbundle By Name(w402) -> ("Step Size"=w411:dbl)
                    n219 = call "Mapping Merge Real Positions v10.2.1.vi"("Live Data In"=w415, "X in (1D)"=w413, "Y in (1D)"=w412, "Step Size"=w411) -> ("Live Data Out"=w414:dbl[][])  [unwired: 11 in]
                    "Full Data" <- w414
                    n220 = call "Export_2DtoTxt v10.6.0.vi"("ITC503 Current Values"=w410, "iHR Current Values"=w409, "CCD Temperature"=w408, "CCD Area"=w405, "CCD ADC"=w404, "CCD Gain"=w403, "Export Type"="Mapping", "Spectra Settings"=w407, "Filename"=w416, "Data (2D)"=w414, "Mapping Parameters"=w402) -> ()  [unwired: 8 in, 1 out]
                  }
                  frame #1 {
                    # "reset indicators"
                    n221 = local write "Start"(FALSE ("Start")) -> ()
                    n222 = local write "CCD Current Rep."("0/0" ("CCD3000 Current Rep.")) -> ()
                    n223 = case shown="False" w418 {
                      frame False {
                        n224 = call "Video Toolset Stop.vi"() -> ()  [unwired: 3 in]
                      }
                      frame True {
                      }
                    }
                    n225 = property on="Measuring" class="Bool (strict)"("BoolText.Text"="" ("Boolescher Text.Text")) -> ()  [unwired: 2 in, 2 out]
                    n226 = property on="Measuring" class="Bool (strict)"("Blinking"=FALSE ("Measuring")) -> ()  [unwired: 2 in, 2 out]
                    n227 = global write "Global Variables.vi" "Mapping Running?"(FALSE ("Mapping Running?")) -> ()
                  }
                }
              }
            }
          }
        }
        n228 = local read "Exit"() -> (w40:bool)
      }
    }
    frame #2 {
      n229 = invoke class="VI Interface Type 0" method="Ctrl Val.Set"(reference=w425, "Control Name"="Exit" ("Elementname"), "Value"=TRUE) -> ()  [unwired: 2 in, 5 out]
      n230 = local read "AutoClose"() -> (w424:bool)
      n231 = flat-sequence {
        tunnel: w424 -> [w428]
        frame #0 {
          # "reset and close"
          n232 = control-ref of="Dieses VI"() -> (w431:refnum<vi>)
          n233 = global write "Global Variables.vi" "Mapping Open?"(FALSE ("Mapping Open?")) -> ()
          n234 = invoke class="VI" method="Default Vals.Reinit All"(reference=w431) -> (reference out=w429:refnum<vi>)  [unwired: 2 in, 2 out]
          n235 = property on="Measuring" class="Bool (strict)"("BoolText.Text"="" ("Boolescher Text.Text")) -> ()  [unwired: 2 in, 2 out]
          n236 = property class="App"() -> ("App.Kind"=w432:T12)  [unwired: 2 in, 2 out]
          n237 = case shown="\"invalid app kind\", Default" w432 {
            tunnel: w429 -> [w434 w436]
            tunnel: w428 -> [_ w435]
            frame "invalid app kind", Default {
              n238 = invoke on="Invoke Node" class="VI" method="FP.Close"(reference=w434) -> ()  [unwired: 2 in, 3 out]
            }
            frame "Development System" {
              n239 = case shown="True" w435 {
                tunnel: w436 -> [_ w437]
                frame False {
                }
                frame True {
                  n240 = invoke on="Invoke Node" class="VI" method="FP.Close"(reference=w437) -> ()  [unwired: 2 in, 3 out]
                }
              }
            }
          }
        }
      }
    }
  }
